vi "Untitled 1.vi"   [LabVIEW 2020]
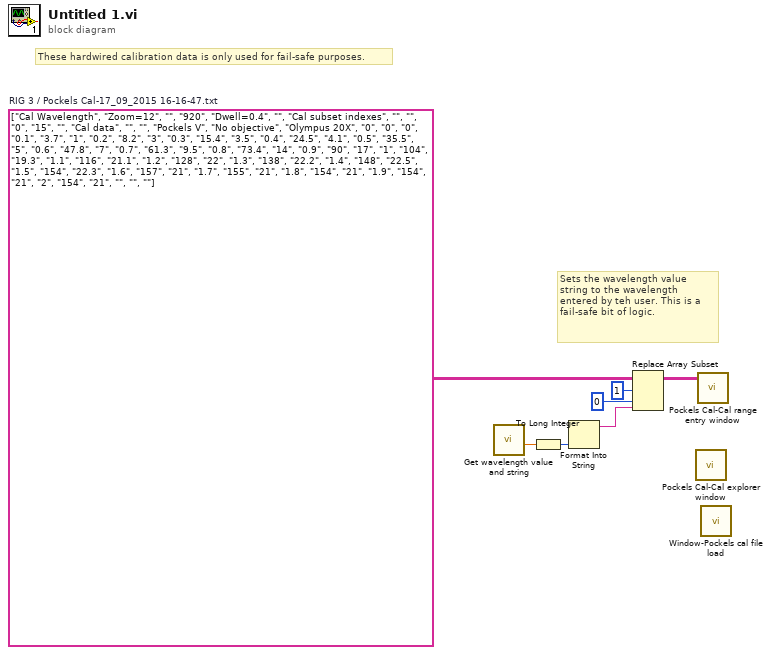
[diagram p0: block diagram]
diagram:
  w7 = string[][] [["Cal Wavelength", "Zoom=12", ""], ["920", "Dwell=0.4", ""], ["Cal subset indexes", "", ""], ["0", "15", ""], ["Cal data", "", ""], ["Pockels V", "No objective", "Olympus 20X"], ["0", "0", "0"], ["0.1", "3.7", "1"], ["0.2", "8.2", "3"], ["0.3", "15.4", "3.5"], ["0.4", "24.5", "4.1"], ["0.5", "35.5", "5"], ["0.6", "47.8", "7"], ["0.7", "61.3", "9.5"], ["0.8", "73.4", "14"], ["0.9", "90", "17"], ["1", "104", "19.3"], ["1.1", "116", "21.1"], ["1.2", "128", "22"], ["1.3", "138", "22.2"], ["1.4", "148", "22.5"], ["1.5", "154", "22.3"], ["1.6", "157", "21"], ["1.7", "155", "21"], ["1.8", "154", "21"], ["1.9", "154", "21"], ["2", "154", "21"], ["", "", ""]]  # RIG 3 / Pockels Cal-17_09_2015 16-16-47.txt
  # "Sets the wavelength value string to the wavelength entered by teh user. This is a fail-safe bit of logic."
  # "These hardwired calibration data is only used for fail-safe purposes."
  n1 = call "Get wavelength value and string.vi"() -> ("Wavelength value"=w6:dbl)  [unwired: 9 in, 2 out]
  n2 = To Long Integer(number=w6) -> (32bit integer=w2:i32)
  n3 = Format Into String(w2) -> (resulting string=w5:string)  [unwired: 3 in, 1 out]
  n4 = Replace Array Subset(array=w7, new element=w5, index (row)=1, index (col)=0 ("disabled index (col)")) -> (w1:string[][])
  n5 = call "Pockels Cal-Cal explorer window.vi"() -> ()  [unwired: 12 in]
  n6 = call "Pockels Cal-Cal range entry window.vi"("Calibration data array (inc. data header row)"=w1) -> ()  [unwired: 9 in, 2 out]
  n7 = call "Window-Pockels cal file load.vi"() -> ()  [unwired: 12 in]
